vi "Launch Nested Actors.vi"(8 "error in (no error)":errorcluster, 10 "Selection UI Subpanel Ref":refnum<vi>, 11 "Pane Relief Main UI in":refnum<class "Pane Relief Main UI.lvclass">) -> (0 "error out":errorcluster, 3 "Pane Relief Main UI out":refnum<class "Pane Relief Main UI.lvclass">)   [LabVIEW 2017, in "Pane Relief Main UI.lvlib" / "Pane Relief Main UI.lvclass"]
uses:
  Pane Relief Main UI.lvclass
  C:/Program Files (x86)/National Instruments/LabVIEW 2017/vi.lib/MNProjects/Panel Manager/panel-actors/Source/Panel Actor/Panel Actor.lvclass
  Splitter Settings UI/Splitter Settings UI/Splitter Settings UI.lvclass
  Instructions UI/Instructions UI/Instructions UI.lvclass
  Panel Object Actions UI/Panel Object Actions UI/Panel Object Actions UI.lvclass
  Pane Settings UI/Pane Settings UI/Pane Settings UI.lvclass
  Pane Relief Main UI.lvclass/Pane Relief Main UI.ctl
  <vilib>/MNProjects/Panel Manager/panel-manager/Source/Panel/Subpanel/Subpanel.lvclass
  C:/Program Files (x86)/National Instruments/LabVIEW 2017/vi.lib/MNProjects/Panel Manager/panel-manager/Source/Panel/Panel.lvclass
  <vilib>/MNProjects/Panel Manager/panel-manager/Source/Panel/Subpanel/Subpanel.vi
  <vilib>/MNProjects/Panel Manager/panel-manager/Source/MGI-Panel Manager.lvlib
  <vilib>/MNProjects/Panel Manager/panel-actors/Source/Panel Actor/Panel Actor.lvclass
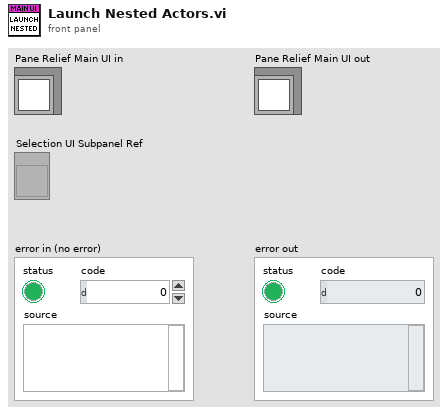
[diagram p1: front panel]
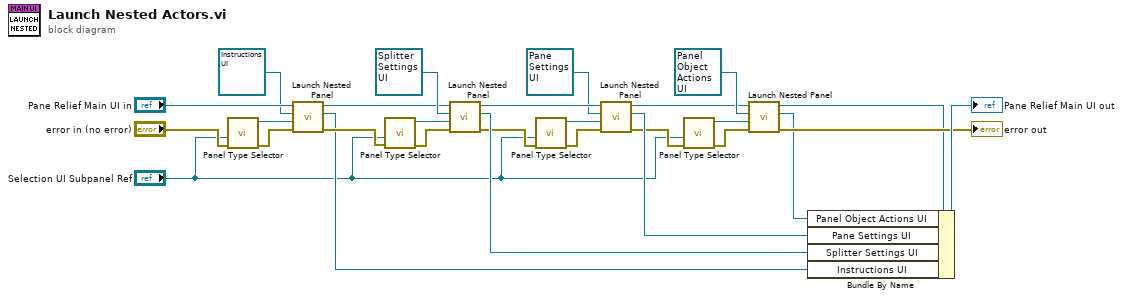
[diagram p0: block diagram]
diagram:
  n1 = call-poly <vilib>:"Panel Type Selector.vi"("Error In"="error in (no error)", "Sub Panel"="Selection UI Subpanel Ref") -> ("Error Out"=w14:errorcluster, "Subpanel Out"=w15:refnum<class "Subpanel.lvclass">)  [unwired: 8 in]
  n2 = call <vilib>:"Launch Nested Panel.vi"("error in (no error)"=w14, "Panel"=w15, "Nested Panel Actor"=refnum<class "Instructions UI.lvclass"> refnum ("Instructions UI.lvlib:Instructions UI.lvclass"), "Panel Actor in"="Pane Relief Main UI in") -> ("error out"=w12:errorcluster, "Nested Actor's Enqueuer"=w10:refnum<class "Message Enqueuer.lvclass">, "Panel Actor out"=w11:refnum<class "Pane Relief Main UI.lvclass">)  [unwired: 4 in, 1 out]
  n3 = call-poly <vilib>:"Panel Type Selector.vi"("Error In"=w12, "Sub Panel"="Selection UI Subpanel Ref") -> ("Error Out"=w19:errorcluster, "Subpanel Out"=w18:refnum<class "Subpanel.lvclass">)  [unwired: 8 in]
  n4 = call <vilib>:"Launch Nested Panel.vi"("error in (no error)"=w19, "Panel"=w18, "Nested Panel Actor"=refnum<class "Splitter Settings UI.lvclass"> refnum ("Splitter Settings UI.lvlib:Splitter Settings UI.lvclass"), "Panel Actor in"=w11) -> ("error out"=w22:errorcluster, "Nested Actor's Enqueuer"=w24:refnum<class "Message Enqueuer.lvclass">, "Panel Actor out"=w21:refnum<class "Pane Relief Main UI.lvclass">)  [unwired: 4 in, 1 out]
  n5 = call-poly <vilib>:"Panel Type Selector.vi"("Error In"=w22, "Sub Panel"="Selection UI Subpanel Ref") -> ("Error Out"=w3:errorcluster, "Subpanel Out"=w4:refnum<class "Subpanel.lvclass">)  [unwired: 8 in]
  n6 = call <vilib>:"Launch Nested Panel.vi"("error in (no error)"=w3, "Panel"=w4, "Nested Panel Actor"=refnum<class "Pane Settings UI.lvclass"> refnum ("Pane Settings UI.lvlib:Pane Settings UI.lvclass"), "Panel Actor in"=w21) -> ("error out"=w6:errorcluster, "Nested Actor's Enqueuer"=w23:refnum<class "Message Enqueuer.lvclass">, "Panel Actor out"=w5:refnum<class "Pane Relief Main UI.lvclass">)  [unwired: 4 in, 1 out]
  n7 = call-poly <vilib>:"Panel Type Selector.vi"("Error In"=w6, "Sub Panel"="Selection UI Subpanel Ref") -> ("Error Out"=w8:errorcluster, "Subpanel Out"=w7:refnum<class "Subpanel.lvclass">)  [unwired: 8 in]
  n8 = call <vilib>:"Launch Nested Panel.vi"("error in (no error)"=w8, "Panel"=w7, "Nested Panel Actor"=refnum<class "Panel Object Actions UI.lvclass"> refnum ("Panel Object Actions UI.lvlib:Panel Object Actions UI.lvclass"), "Panel Actor in"=w5) -> ("error out"=→"error out":errorcluster, "Nested Actor's Enqueuer"=w16:refnum<class "Message Enqueuer.lvclass">, "Panel Actor out"=w17:refnum<class "Pane Relief Main UI.lvclass">)  [unwired: 4 in, 1 out]
  n9 = Bundle By Name(cluster=w17, "Panel Object Actions UI"=w16, "Pane Settings UI"=w23, "Splitter Settings UI"=w24, "Instructions UI"=w10) -> (→"Pane Relief Main UI out":refnum<class "Pane Relief Main UI.lvclass">)
